vi "mode initial.vi"(8 "错误输入（无错误）":errorcluster, 11 "引用句柄输入":refnum<k21>) -> (0 "Error Out":errorcluster)   [LabVIEW 2017]
uses:
  <vilib>/VirtualBench/VirtualBench.lvlib
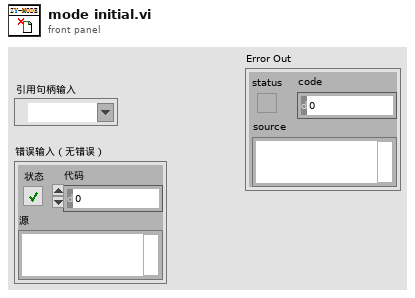
[diagram p1: front panel]
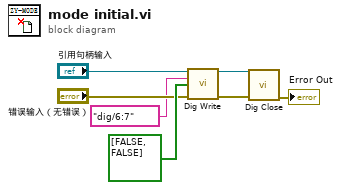
[diagram p0: block diagram]
diagram:
  n1 = call <vilib>:"Dig Write.vi"("Instrument Handle In"="引用句柄输入", "Lines"=tag "dig/6:7", "Data"=bool[] [FALSE, FALSE], "Error In"="错误输入（无错误）") -> ("Instrument Handle Out"=w6:refnum<k21>, "Error Out"=w7:errorcluster)  [unwired: 10 in]
  n2 = call <vilib>:"Dig Close.vi"("Instrument Handle In"=w6, "Error In"=w7) -> ("Error Out"=→"Error Out":errorcluster)  [unwired: 13 in]
